vi "Drive Easy.vi"(4 "D Gain":dbl=5e-05 format="%#_13g", 6 "P Gain":dbl=0.0725 format="%#_13g", 7 "Automatic Drive Stright Range":dbl, 8 "Operator":dbl, 9 "Buttons":bool[](array[boolean]), 10 "Axes":dbl[](array[numeric]), 11 "Get All":T2 {"Calibration"."CurrentMode" items=["BootTareGryoAccel"=0, "Temperature"=1, "Magnetometer12Pt"=2, "Magnetometer360"=3, "Accelerometer"=5]}) -> (2 "Left Motor Value":dbl, 3 "Right Motor Value":dbl, 5 "Control Mode":T1)   [LabVIEW 2016]
uses:
  <vilib>/Rock Robotics/WPI/ThirdParty/Sensors/Pigeon IMU/CTRE_PigeonIMU_GlobalStatus.ctl
  <vilib>/Rock Robotics/WPI/ThirdParty/Sensors/Pigeon IMU/CTRE_PigeonIMU_PigeonState.ctl
  <vilib>/Rock Robotics/WPI/ThirdParty/Sensors/Pigeon IMU/CTRE_PigeonIMU_CalibrationMode.ctl
  <vilib>/Rock Robotics/WPI/ThirdParty/CanMotor/TalonSRX/WPI_CANTalonSRX_APIControlMode.ctl
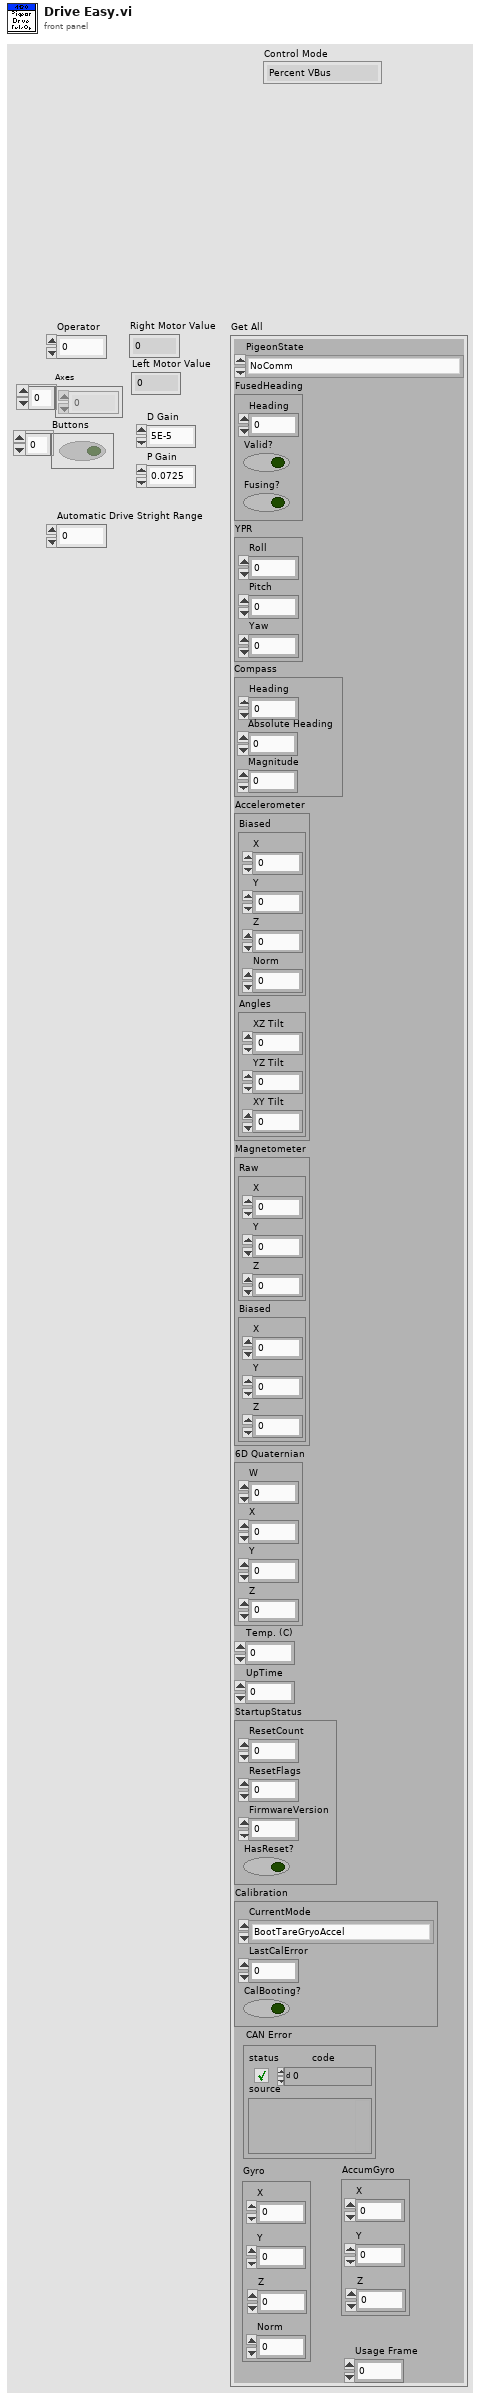
[diagram p1: front panel]
types:
  T1 = typedef "WPI_CANTalonSRX_APIControlMode.ctl" = enum8{"Percent VBus", "Speed", "Position", "Slave", "Unchanged / Invalid", "Voltage Compensation", "Current", "Motion Profile", "Motion Magic"}
  T2 = typedef "CTRE_PigeonIMU_GlobalStatus.ctl" = cluster{"PigeonState":T3, "FusedHeading":cluster{"Heading":dbl, "Valid?":bool, "Fusing?":bool}, "YPR":cluster{"Yaw":dbl, "Pitch":dbl, "Roll":dbl}, "Compass":cluster{"Heading":dbl, "Magnitude":dbl, "Absolute Heading":dbl}, "Accelerometer":cluster{"Biased":cluster{"X":i16, "Y":i16, "Z":i16, "Norm":i16}, "Angles":cluster{"XZ Tilt":dbl, "YZ Tilt":dbl, "XY Tilt":dbl}}, "Magnetometer":cluster{"Raw":cluster{"X":i16, "Y":i16, "Z":i16}, "Biased":cluster{"X":i16, "Y":i16, "Z":i16}}, "Gyro":cluster{"X":dbl, "Y":dbl, "Z":dbl, "Norm":dbl}, "6D Quaternian":cluster{"W":dbl, "X":dbl, "Y":dbl, "Z":dbl}, "Temp. (C)":dbl, "UpTime":u32, "StartupStatus":cluster{"ResetCount":i32, "ResetFlags":i32, "FirmwareVersion":i32, "HasReset?":bool}, "Calibration":cluster{"CurrentMode":T4, "LastCalError":i32, "CalBooting?":bool}, "CAN Error":errorcluster, "AccumGyro":cluster{"X":dbl, "Y":dbl, "Z":dbl}, "Usage Frame":u32}
  T3 = typedef "CTRE_PigeonIMU_PigeonState.ctl" = enum16{"NoComm", "Initializing", "Ready", "UserCalibration"}
  T4 = typedef "CTRE_PigeonIMU_CalibrationMode.ctl" = u16
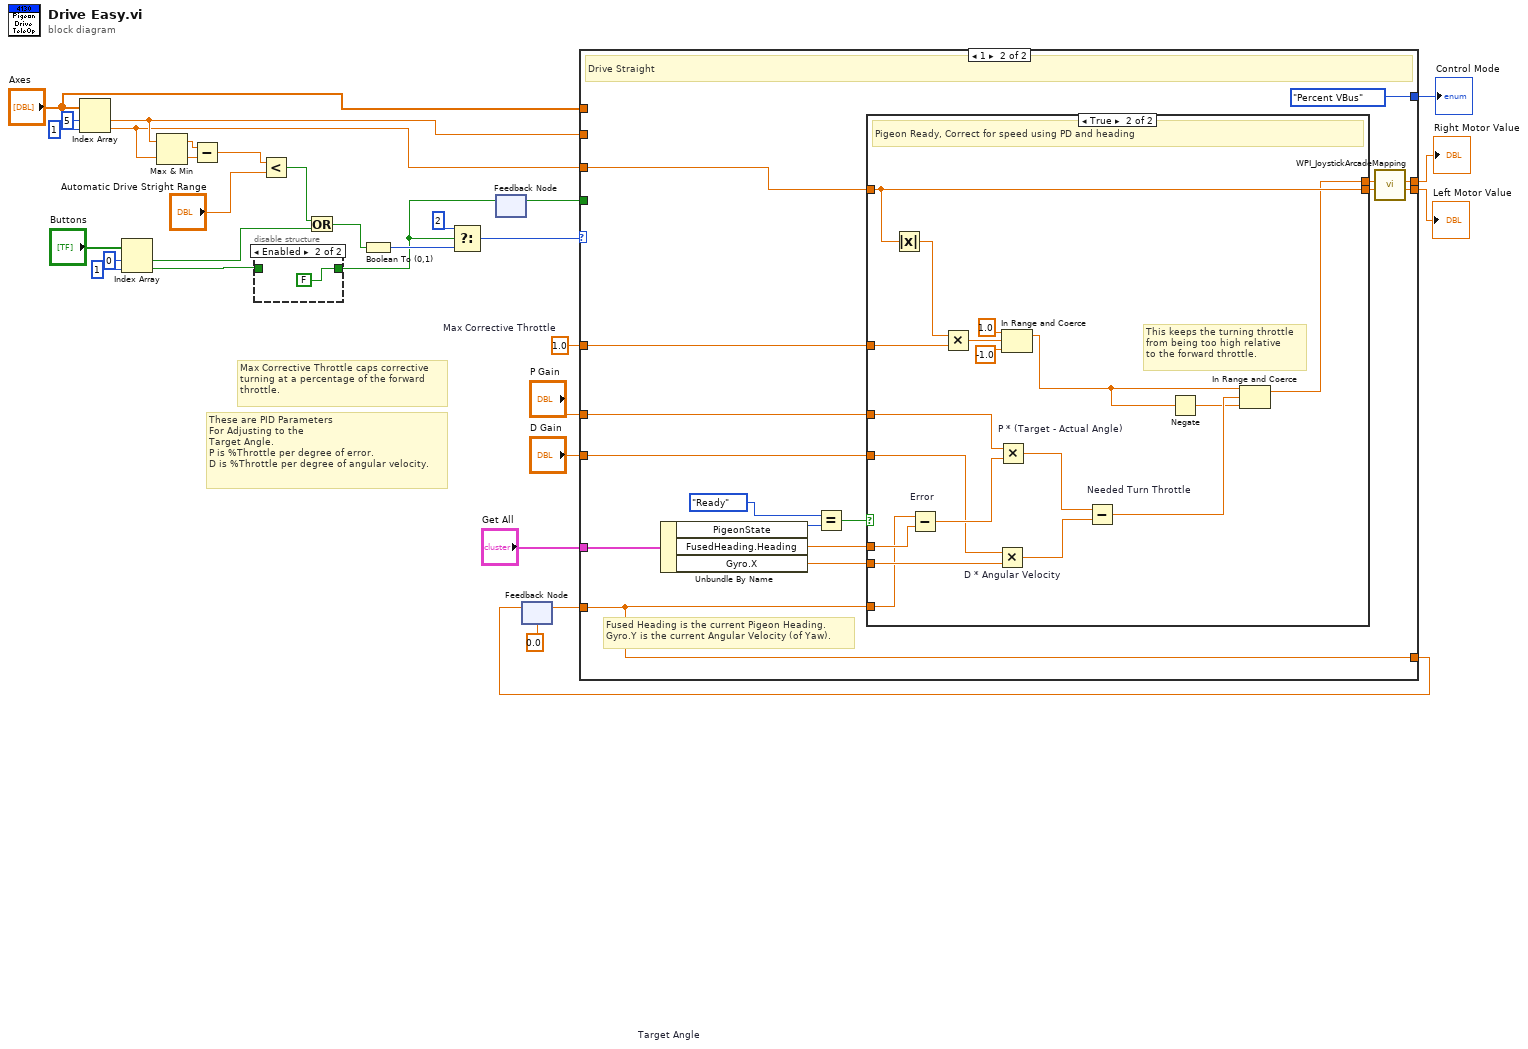
[diagram p0: block diagram]
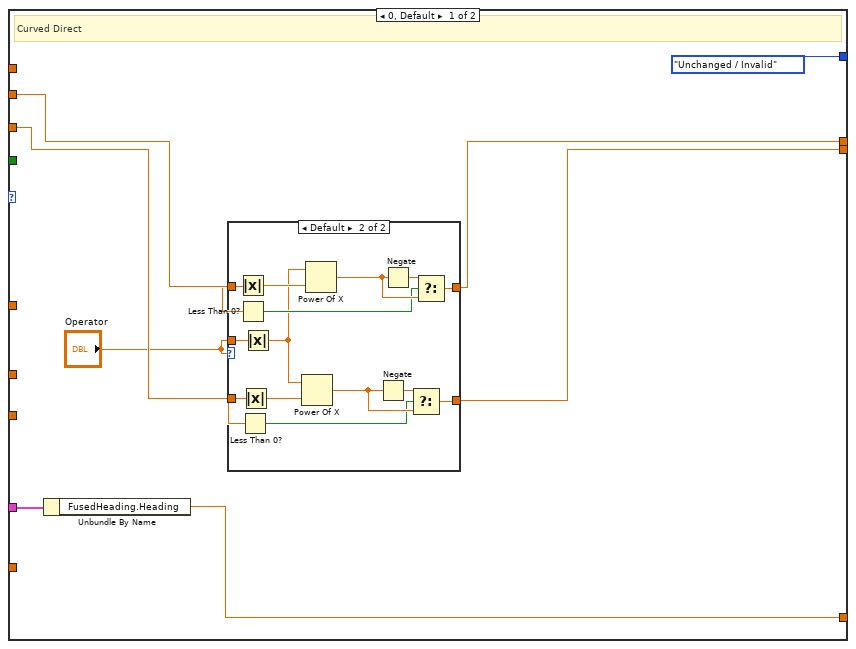
[diagram p3: hidden frame]
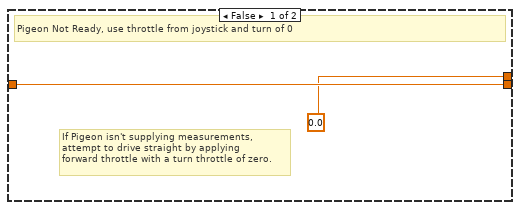
[diagram p5: hidden frame]
diagram:
  w28 = 1.0  # Max Corrective Throttle
  # "Max Corrective Throttle caps corrective\nturning at a percentage of the forward\nthrottle."
  # "These are PID Parameters\nFor Adjusting to the\nTarget Angle.\nP is %Throttle per degree of error.\nD is %Throttle per degree of angular velocity."
  n1 = Index Array(array="Axes", index #1=5 ("index"), index #2=1 ("index")) -> (element #1=w7:dbl, element #2=w6:dbl)
  n2 = Index Array(array="Buttons", index #1=0 ("index"), index #2=1 ("index")) -> (element #1=w10:bool, element #2=w12:bool)
  n3 = Max & Min(x=w7, y=w6) -> (max(x,y)=w5:dbl, min(x,y)=w4:dbl)
  n4 = Subtract(x=w5, y=w4) -> (x-y=w3:dbl)
  n5 = disable-structure shown="Enabled" {
    disable-tunnel: w12 -> [w32 _]
    disable-tunnel: [w32 FALSE] -> w11
    frame Disabled {
    }
    frame Enabled {
    }
  }
  n6 = Less?(x=w3, y="Automatic Drive Stright Range") -> (x < y?=w2:bool)
  n7 = Or(x=w2, y=w10) -> (x .or. y?=w9:bool)
  n8 = Boolean To (0,1)(Boolean=w9) -> (0, 1=w18:i16)
  n9 = Select(t=i16 2, s=w11, f=w18) -> (s? t:f=w17:i16)
  n10 = feedback #1() -> (w13:bool)  [unwired: 1 in]
  n11 = feedback-in #1(w11) -> ()
  n12 = feedback #2 "Target Angle"(0.0 ("Heading")) -> (w29:dbl)
  n13 = case shown="1" w17 {
    tunnel: w7 -> [w38 _]
    tunnel: w6 -> [w37 w72]
    tunnel: "P Gain" -> [_ w67]
    tunnel: "D Gain" -> [_ w66]
    tunnel: [w41 w59] -> w27
    tunnel: w29 -> [_ w59]
    tunnel: w28 -> [_ w65]
    tunnel: [w36 w62] -> w26
    tunnel: [w35 w61] -> w25
    tunnel: "Get All" -> [w40 w60]
    tunnel: [WPI_CANTalonSRX_APIControlMode."Unchanged / Invalid" ("Control Mode") WPI_CANTalonSRX_APIControlMode."Percent VBus" ("Control Mode")] -> w19
    tunnel: "Axes" -> [_ _]
    tunnel: w13 -> [_ _]
    frame 0, Default {
      # "Curved Direct"
      n14 = Unbundle By Name(w40) -> ("FusedHeading.Heading"=w41:dbl)
      n15 = case shown="Default" "Operator" {
        tunnel: [w43 w56] -> w36
        tunnel: [w42 w51] -> w35
        tunnel: w37 -> [w42 w50]
        tunnel: w38 -> [w43 w48]
        tunnel: "Operator" -> [_ w45]
        frame 0 {
        }
        frame Default {
          n16 = Absolute Value(x=w48) -> (abs(x)=w49:dbl)
          n17 = Less Than 0?(x=w48) -> (x < 0?=w47:bool)
          n18 = Less Than 0?(x=w50) -> (x < 0?=w46:bool)
          n19 = Absolute Value(x=w50) -> (abs(x)=w57:dbl)
          n20 = Absolute Value(x=w45) -> (abs(x)=w44:dbl)
          n21 = Power Of X(1:w57, 2:w44) -> (0:w52:dbl)
          n22 = Power Of X(1:w49, 2:w44) -> (0:w54:dbl)
          n23 = Negate(x=w52) -> (-x=w53:dbl)
          n24 = Negate(x=w54) -> (-x=w55:dbl)
          n25 = Select(t=w53, s=w46, f=w52) -> (s? t:f=w51:dbl)
          n26 = Select(t=w55, s=w47, f=w54) -> (s? t:f=w56:dbl)
        }
      }
    }
    frame 1 {
      # "Fused Heading is the current Pigeon Heading.\nGyro.Y is the current Angular Velocity (of Yaw)."
      # "Drive Straight"
      n27 = Unbundle By Name(w60) -> ("PigeonState"=w70:T3, "FusedHeading.Heading"=w69:dbl, "Gyro.X"=w68:dbl)
      n28 = Equal?(x=CTRE_PigeonIMU_PigeonState."Ready" ("PigeonState"), y=w70) -> (x = y?=w73:bool)
      n29 = case shown="True" w73 {
        tunnel: w72 -> [w75 w84]
        tunnel: [w75 w84] -> w63
        tunnel: [0.0 ("upper limit") w77] -> w64
        tunnel: w69 -> [_ w93]
        tunnel: w59 -> [_ w76]
        tunnel: w68 -> [_ w90]
        tunnel: w67 -> [_ w91]
        tunnel: w66 -> [_ w89]
        tunnel: w65 -> [_ w86]
        frame False {
          # "If Pigeon isn't supplying measurements,\nattempt to drive straight by applying\nforward throttle with a turn throttle of zero."
          # "Pigeon Not Ready, use throttle from joystick and turn of 0"
        }
        frame True {
          # "This keeps the turning throttle\nfrom being too high relative\nto the forward throttle."
          # "Pigeon Ready, Correct for speed using PD and heading"
          n30 = Absolute Value(x=w84) -> (abs(x)=w85:dbl)
          n31 = Subtract "Error"(x=w76, y=w93) -> (x-y=w92:dbl)
          n32 = Multiply ("P * (Target - Actual Angle)")(x=w85, y=w86) -> (x*y=w81:dbl)
          n33 = Multiply "D * Angular Velocity"(x=w89, y=w90) -> (x*y=w87:dbl)
          n34 = Multiply "P * (Target - Actual Angle)"(x=w91, y=w92) -> (x*y=w88:dbl)
          n35 = In Range and Coerce(upper limit=1.0, x=w81, lower limit=-1.0) -> (coerced(x)=w79:dbl)  [unwired: 1 out]
          n36 = Subtract "Needed Turn Throttle"(x=w88, y=w87) -> (x-y=w80:dbl)
          n37 = Negate(x=w79) -> (-x=w78:dbl)
          n38 = In Range and Coerce(upper limit=w79, x=w80, lower limit=w78) -> (coerced(x)=w77:dbl)  [unwired: 1 out]
        }
      }
      n39 = call <vilib>:"WPI_JoystickArcadeMapping.vi"("Y axis value"=w63, "X axis value"=w64) -> ("Right Motor Value"=w61:dbl, "Left Motor Value"=w62:dbl)  [unwired: 8 in]
    }
  }
  "Right Motor Value" <- w26
  "Left Motor Value" <- w25
  "Control Mode" <- w19
  n40 = feedback-in #2(w27) -> ()
